vi "fibonnacci.vi"() -> ()   [LabVIEW 2021]
panel:
  out "Array 2":i32[](array[numeric])
  out "Array":dbl[](array[numeric])
  in  "Numeric 4":dbl
  out "Numeric 2":dbl
  out "Numeric":dbl
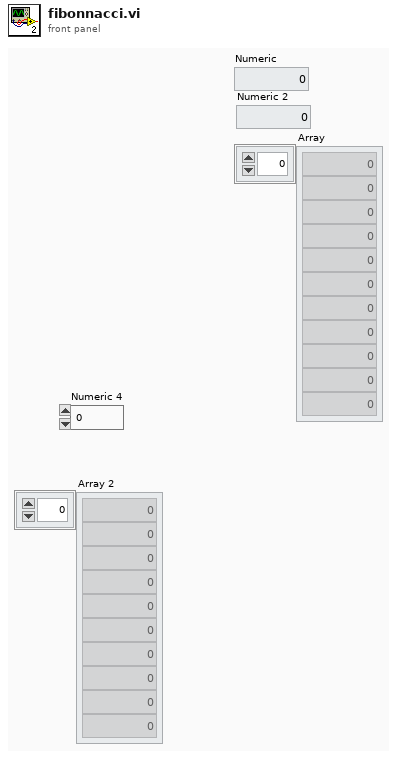
[diagram p1: front panel]
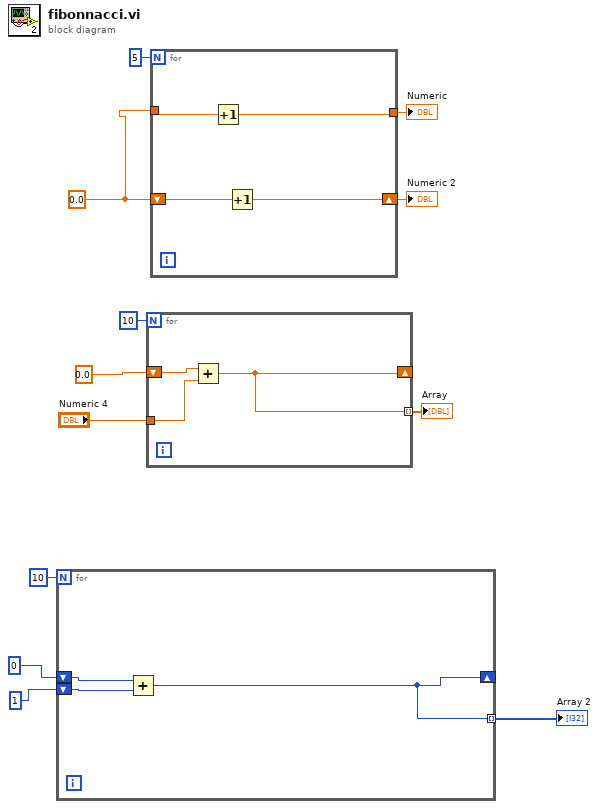
[diagram p0: block diagram]
diagram:
  w11 = 0.0
  n1 = for {
    N: 10 -> [_]
    shift-right: [w14] -> _
    shift-left: 0 -> [w15]
    tunnel: [w14] -> w2 mode=indexing
    shift-left: 1 -> [w13]
    n2 = Add(x=w15, y=w13) -> (x+y=w14:i32)
  }
  "Array 2" <- w2
  n3 = for {
    N: 10 -> [_]
    shift-right: [w16] -> _
    shift-left: 0.0 -> [w18]
    tunnel: "Numeric 4" -> [w17]
    tunnel: [w16] -> w5 mode=indexing
    n4 = Add(x=w18, y=w17) -> (x+y=w16:dbl)
  }
  "Array" <- w5
  n5 = for {
    N: 5 -> [_]
    shift-right: [w22] -> w9
    shift-left: w11 -> [w21]
    tunnel: w11 -> [w20]
    tunnel: [w19] -> w10
    n6 = Increment(x=w20) -> (x+1=w19:dbl)
    n7 = Increment(x=w21) -> (x+1=w22:dbl)
  }
  "Numeric" <- w10
  "Numeric 2" <- w9
